vi "ep_NEMA Unbalance (3-Phases).vi"(8 "error in (no error)":errorcluster, 11 "voltage RMS values (3-phases)":dbl[](array[numeric])) -> (0 "error out":errorcluster, 2 "unbalance derating factor":dbl, 3 "unbalance [%]":dbl)   [LabVIEW 2014, in "NI_EP_Motor Monitoring.lvlib"]
uses:
  <vilib>/addons/Electrical Power/Motor Monitoring/NI_EP_Motor Monitoring.lvlib
  <vilib>/Analysis/baseanly.llb/Mean (DBL).vi
  <vilib>/Analysis/NI_AALBase.lvlib
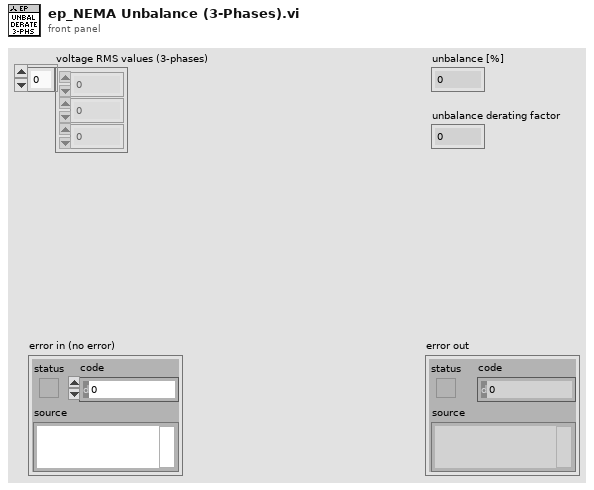
[diagram p1: front panel]
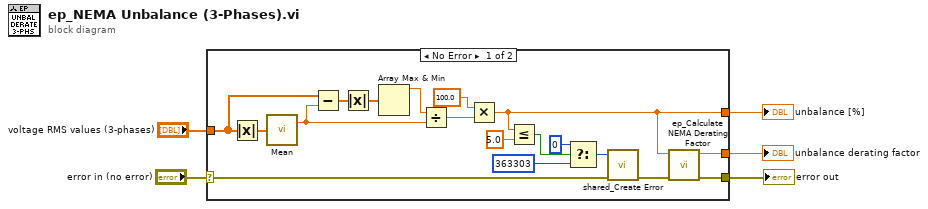
[diagram p0: block diagram]
diagram:
  n1 = case shown="No Error" "error in (no error)" {
    selector: "error in (no error)" -> [w12 w24]
    tunnel: [w23 _] -> w5
    tunnel: [w7 _] -> w4
    tunnel: "voltage RMS values (3-phases)" -> [w19 _]
    tunnel: [w18 w24] -> w1
    frame No Error {
      n2 = Absolute Value(x=w19) -> (abs(x)=w9:dbl[])
      n3 = call-poly <vilib>:"Mean.vi"("X"=w9) -> ("mean"=w10:dbl)  [unwired: 1 out]
      n4 = Subtract(x=w19, y=w10) -> (x-y=w20:dbl[])
      n5 = Absolute Value(x=w20) -> (abs(x)=w21:dbl[])
      n6 = Array Max & Min(array=w21) -> (max value=w22:dbl)  [unwired: 3 out]
      n7 = Divide(x=w22, y=w10) -> (x/y=w8:dbl)
      n8 = Multiply(x=100.0 ("y"), y=w8) -> (x*y=w7:dbl)
      n9 = Less Or Equal?(x=w7, y=5.0) -> (x <= y?=w17:bool)
      n10 = Select(t=0 ("error code (0)"), s=w17, f=363303 ("error code (0)")) -> (s? t:f=w13:i32)
      n11 = call <vilib>:"shared_Create Error.vi"("error in (no error)"=w12, "error code (0)"=w13) -> ("error out"=w11:errorcluster)  [unwired: 9 in]
      n12 = call <vilib>:"ep_Calculate NEMA Derating Factor.vi"("error in (no error)"=w11, "NEMA unbalance [%]"=w7) -> ("error out"=w18:errorcluster, "NEMA unbalance derating factor"=w23:dbl)  [unwired: 8 in]
    }
    frame Error {
    }
  }
  "unbalance derating factor" <- w5
  "unbalance [%]" <- w4
  "error out" <- w1
